vi "Traffic Light Control - ENUM & Case Structure.vi"() -> ()   [LabVIEW 2016]
panel:
  in  "Selelct":enum16{"Red", "Yellow", "Green"}(ring)
  out "Boolean 3":bool
  out "Boolean 2":bool
  out "Boolean":bool
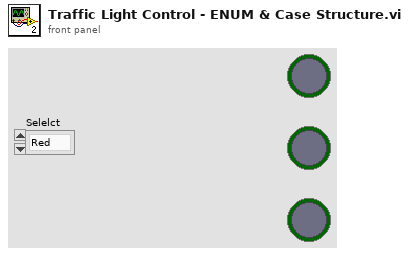
[diagram p1: front panel]
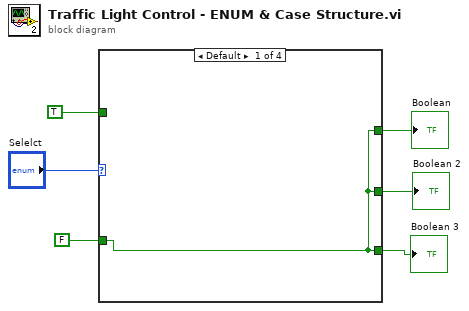
[diagram p0: block diagram]
diagram:
  n1 = case shown="Default" "Selelct" {
    tunnel: [w7 w8 w11 w13] -> w6
    tunnel: FALSE -> [w7 w8 w11 w12]
    tunnel: [w7 w9 w11 w12] -> w4
    tunnel: [w7 w8 w10 w12] -> w3
    tunnel: TRUE -> [_ w9 w10 w13]
    frame Default {
    }
    frame "Red" {
    }
    frame "Yellow" {
    }
    frame "Green" {
    }
  }
  "Boolean" <- w4
  "Boolean 2" <- w3
  "Boolean 3" <- w6
